vi "Manual Control - Sensors Port (SubVI).vi"(8 "error in (no error)":errorcluster, 11 "Machine Name":string) -> (0 "error out":errorcluster, 3 "Sensor Port":i32)   [LabVIEW 2019]
uses:
  Controls/FGV States.ctl
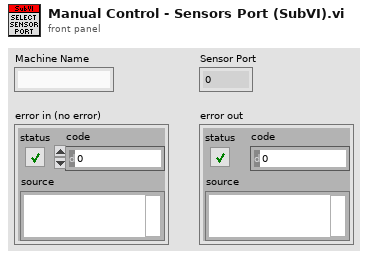
[diagram p1: front panel]
types:
  T1 = typedef "FGV States.ctl" = enum16{"Read", "Write"}
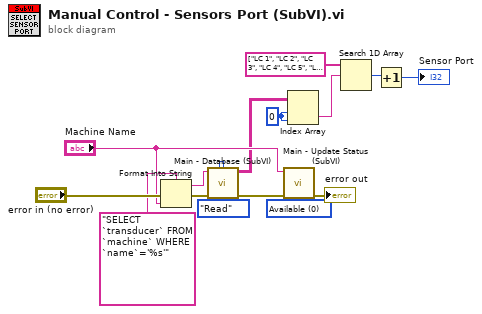
[diagram p0: block diagram]
diagram:
  w10 = u16 0 items=["Available", "Running"] ("Status")
  w7 = 0 ("index (row)")
  n1 = Format Into String(format string="SELECT `transducer` FROM `machine` WHERE `name`='%s'" ("source"), error in="error in (no error)", "Machine Name") -> (resulting string=w5:string, error out=w4:errorcluster)  [unwired: 1 in]
  n2 = call "Main - Database (SubVI).vi"("Enum"=FGV_States."Read", "error in (no error)"=w4, "SQL query"=w5) -> ("error out"=w11:errorcluster, "data"=w8:string[][])  [unwired: 7 in]
  n3 = call "Main - Update Status (SubVI).vi"("Status"=w10, "error in"=w11, "Machine Name"="Machine Name") -> ("error out"=→"error out":errorcluster)  [unwired: 8 in]
  n4 = Index Array(array=w8, index (row)=w7, index (col)=w7) -> (element=w9:string)
  n5 = Search 1D Array(1D array=string[] ["LC 1", "LC 2", "LC 3", "LC 4", "LC 5", "LC 6", "LC 7", "LC 8", "TD 1", "TD 2", "TD 3", "TD 4", "TD 5", "TD 6", "TD 7", "TD 8", "TD 9", "TD 10", "TD 11", "TD 12"], element=w9) -> (index of element=w2:i32)  [unwired: 1 in]
  n6 = Increment(x=w2) -> (x+1=→"Sensor Port":i32)
